vi "Handle Last Ack Core.vi"(4 "error in (no error)":errorcluster, 6 "Last Ack":refnum<class "Last Ack.lvclass">, 7 "WebSocket Server in":refnum<class "WebSocket Server.lvclass">) -> (0 "error out":errorcluster, 3 "WebSocket Server out":refnum<class "WebSocket Server.lvclass">)   [LabVIEW 2021, in "WebSocket Actors.lvlib" / "WebSocket Server.lvclass"]
doc: "(<B>Filename</B>: Actor Framework.lvlib:Actor.lvclass:Handle Last Ack Core.vi)\n\nDefines how the caller actor responds to the Last Ack message from a nested actor. The Last Ack message is the final message a nested actor sends to its caller before it shuts down. The message contains information about the final state of the nested actor.\n\nBy default, this method does nothing except return any error the nested actor sent. A descendant class may override this method to define behavior."
uses:
  WebSocket Server.lvclass
  <vilib>/ActorFramework/LastAck/Last Ack.lvclass
  WebSocket Service/WebSocket Service.lvclass
  <vilib>/ActorFramework/LastAck/Last Ack.lvclass/Last Ack.ctl
  WebSocket Service/WebSocket Service.lvclass/WebSocket Service.ctl
  WebSocket Server.lvclass/WebSocket Server.ctl
  WebSocket Service/properties/Read Service Name.vi
  <vilib>/ActorFramework/Actor/Actor.lvclass
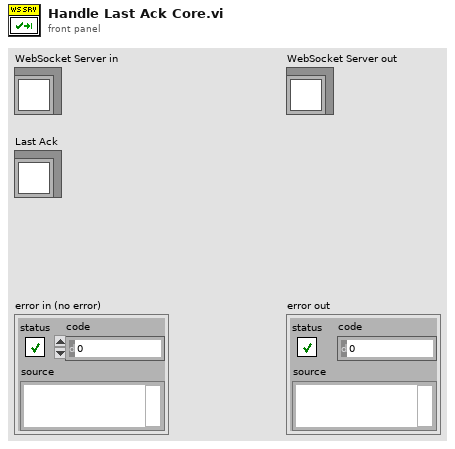
[diagram p1: front panel]
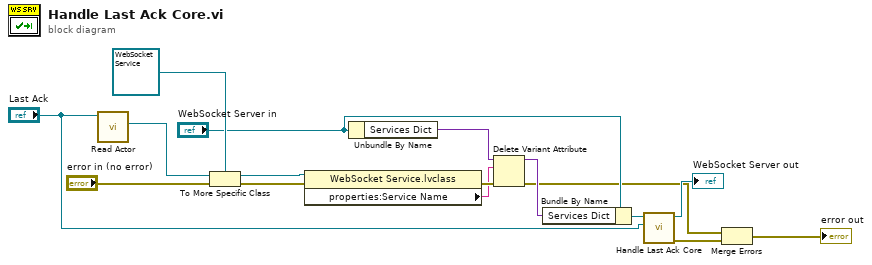
[diagram p0: block diagram]
diagram:
  n1 = call <vilib>:"Read Actor.vi"("Last Ack"="Last Ack") -> ("Actor"=w15:refnum<class "Actor.lvclass">)  [unwired: 10 in]
  n2 = To More Specific Class(target class=refnum<class "WebSocket Service.lvclass"> refnum ("WebSocket Actors.lvlib:WebSocket Service.lvclass"), reference=w15, error in="error in (no error)") -> (specific class reference=w13:refnum<class "WebSocket Service.lvclass">, error out=w11:errorcluster)
  n3 = property class="WebSocket Service.lvclass"(reference=w13, error in=w11) -> (error out=w9:errorcluster, "properties:Service Name"=w7:string)  [unwired: 1 out]
  n4 = Unbundle By Name("WebSocket Server in") -> ("Services Dict"=w8:variant)
  n5 = Delete Variant Attribute(4:w9, 6:w7, 7:w8) -> (0:w1:errorcluster, 3:w5:variant)  [unwired: 1 out]
  n6 = Bundle By Name(cluster="WebSocket Server in", "Services Dict"=w5) -> (w4:refnum<class "WebSocket Server.lvclass">)
  n7 = call-parent "Handle Last Ack Core.vi"("Last Ack"="Last Ack", "Actor in"=w4) -> ("error out"=w2:errorcluster, "Actor out"=→"WebSocket Server out":refnum<class "WebSocket Server.lvclass">)  [unwired: 4 in]
  n8 = Merge Errors(w1, w2) -> (→"error out":errorcluster)
